vi "Auto Index_binding.vi"(10 "Recipes.Binding":T1(array[cluster])) -> (2 "Array":T2(array[cluster]))   [LabVIEW 2014]
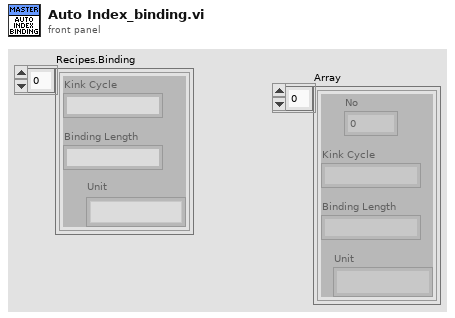
[diagram p1: front panel]
types:
  T1 = cluster{"Kink Cycle":string, "Binding Length":string, "Unit":string}[]
  T2 = cluster{"No":dbl, "Kink Cycle":string, "Binding Length":string, "Unit":string}[]
  T3 = cluster{"No":dbl, "Kink Cycle":string, "Binding Length":string, "Unit":string}
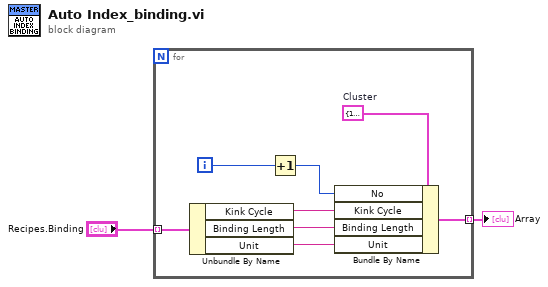
[diagram p0: block diagram]
diagram:
  n1 = for {
    tunnel: "Recipes.Binding" -> [w10] mode=indexing
    tunnel: [w6] -> w2 mode=indexing
    i -> [w4]
    w5 = T3 {"No"=1.0, "Kink Cycle"="", "Binding Length"="", "Unit"="mm"}  # Cluster
    n2 = Unbundle By Name(w10) -> ("Kink Cycle"=w9:string, "Binding Length"=w8:string, "Unit"=w7:string)
    n3 = Increment(x=w4) -> (x+1=w3:i32)
    n4 = Bundle By Name(cluster=w5, "No"=w3, "Kink Cycle"=w9, "Binding Length"=w8, "Unit"=w7) -> (w6:T3)
  }
  "Array" <- w2
